vi "Validate file name.vi"(11 "standard output in":string) -> (1 "No log found":bool, 3 "Log File Name":string)   [LabVIEW 2023, in "VeriStand Console.lvlib"]
uses:
  VeriStand Console.lvlib
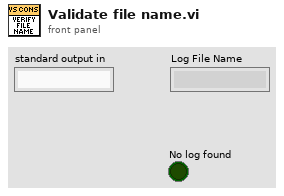
[diagram p1: front panel]
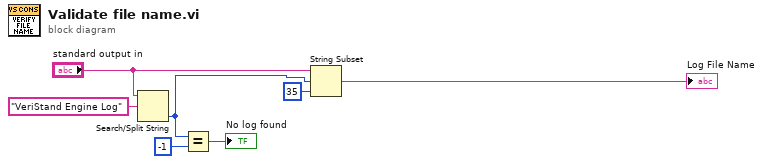
[diagram p0: block diagram]
diagram:
  n1 = Search/Split String(string="standard output in", search string/char (-)="VeriStand Engine Log") -> (offset of match=w3:i32)  [unwired: 1 in, 2 out]
  n2 = Equal?(x=w3, y=-1) -> (x = y?=→"No log found":bool)
  n3 = String Subset(string="standard output in", offset (0)=w3, length (rest)=35 ("length (rest)")) -> (substring=→"Log File Name":string)
